vi "获取平行样数据.vi"(11 "站号":u16(ring)=3 items=["总磷"=1, "总氮"=2, "氨氮"=3, "CODMn"=21, "CODcr"=22, "氟化物"=50]) -> (3 "测量数据区":T1)   [LabVIEW 2016, in "质控单元V4.lvlib"]
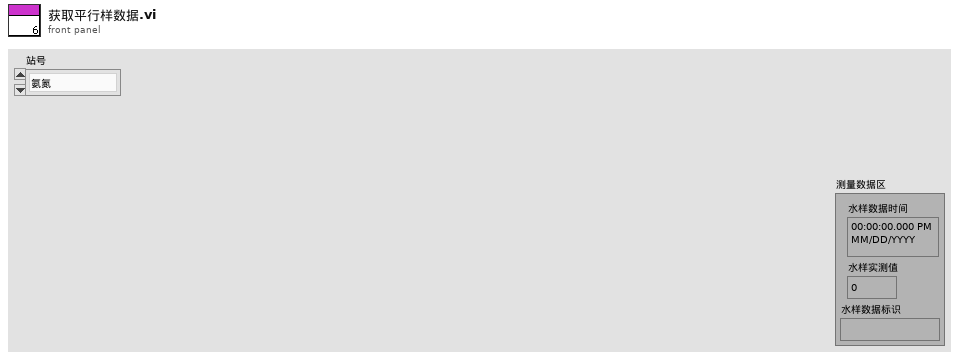
[diagram p1: front panel]
types:
  T1 = cluster{"水样数据时间":timestamp, "水样实测值":sgl, "水样数据标识":string}
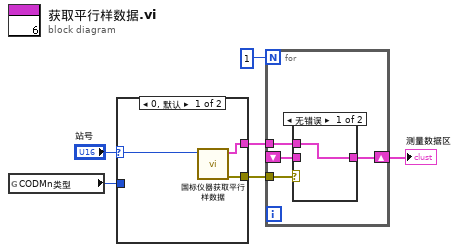
[diagram p0: block diagram]
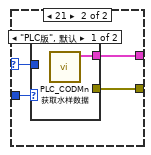
[diagram p3: hidden frame]
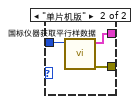
[diagram p4: hidden frame]
diagram:
  n1 = global read "系统交互.vi" "CODMn类型"() -> (w5:enum16{"PLC版", "单片机版"})
  n2 = case shown="0, 默认" "站号" {
    selector: "站号" -> [w9 w11]
    tunnel: [w8 w12] -> w4
    tunnel: w5 -> [_ w13]
    tunnel: [w7 w10] -> w3
    frame 0, Default {
      n3 = call "国标仪器获取平行样数据.vi"("站号"=w9) -> ("error out"=w7:errorcluster, "测量数据区"=w8:T1)  [unwired: 9 in]
    }
    frame 21 {
      n4 = case shown="\"PLC版\", 默认" w13 {
        tunnel: [w14 w17] -> w12
        tunnel: w11 -> [_ w16]
        tunnel: [_ w15] -> w10
        frame "PLC版", Default {
          n5 = call "PLC_CODMn 获取水样数据.vi"() -> ("测量数据区"=w14:T1)  [unwired: 11 in]
        }
        frame "单片机版" {
          n6 = call "国标仪器获取平行样数据.vi"("站号"=w16) -> ("error out"=w15:errorcluster, "测量数据区"=w17:T1)  [unwired: 9 in]
        }
      }
    }
  }
  n7 = for {
    N: 1 -> [_]
    tunnel: w4 -> [w20]
    tunnel: w3 -> [w21]
    shift-right: [w19] -> w1
    shift-left: _ -> [w18]
    n8 = case shown="无错误" w21 {
      tunnel: w20 -> [w22 _]
      tunnel: [w22 w23] -> w19
      tunnel: w18 -> [_ w23]
      frame No Error {
      }
      frame Error {
      }
    }
  }
  "测量数据区" <- w1
